vi "End Drag Nodes.vi"(0 "FSM in":refnum<class "FSM.Graph.lvclass">, 11 "error in (no error)":errorcluster) -> (4 "FSM out":refnum<class "FSM.Graph.lvclass">, 15 "error out":errorcluster)   [LabVIEW 2015, in "FSM.Graph.lvclass"]
uses:
  FSM.Graph.lvclass
  FSM.Graph.lvclass/FSM.Graph.ctl
  FSM.Node/FSM.Node.lvclass
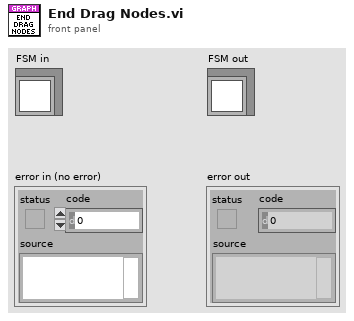
[diagram p1: front panel]
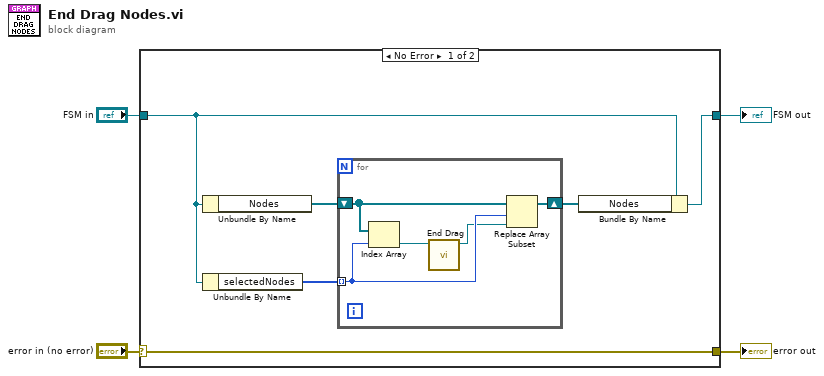
[diagram p0: block diagram]
diagram:
  n1 = case shown="No Error" "error in (no error)" {
    selector: "error in (no error)" -> [w10 w17]
    tunnel: [w10 w17] -> w3
    tunnel: [w6 w16] -> w1
    tunnel: "FSM in" -> [w9 w16]
    frame No Error {
      n2 = Unbundle By Name(w9) -> ("Nodes"=w7:refnum<class "FSM.Node.lvclass">[])
      n3 = Unbundle By Name(w9) -> ("selectedNodes"=w8:i32[])
      n4 = for {
        tunnel: w8 -> [w13] mode=indexing
        shift-right: [w15] -> w5
        shift-left: w7 -> [w14]
        n5 = Index Array(array=w14, index=w13) -> (element=w12:refnum<class "FSM.Node.lvclass">)
        n6 = call "End Drag.vi"("FSM in"=w12) -> ("FSM out"=w11:refnum<class "FSM.Node.lvclass">)  [unwired: 9 in, 1 out]
        n7 = Replace Array Subset(array=w14, new element=w11, index=w13) -> (w15:refnum<class "FSM.Node.lvclass">[])
      }
      n8 = Bundle By Name(cluster=w9, "Nodes"=w5) -> (w6:refnum<class "FSM.Graph.lvclass">)
    }
    frame Error {
    }
  }
  "error out" <- w3
  "FSM out" <- w1
